vi "Intensity Graph Linecut (Horizontal).vi"(8 "error in (no error)":errorcluster, 9 "width (horizontal)":dbl, 11 "graph_utilities in":refnum<class "graph_utilities.lvclass">) -> (0 "error out":errorcluster, 3 "graph_utilities out":refnum<class "graph_utilities.lvclass">)   [LabVIEW 2016, in "graph_utilities.lvclass"]
uses:
  graph_utilities.lvclass
  <vilib>/Analysis/baseanly.llb/A x Vector.vi
  <vilib>/Analysis/NI_AALBase.lvlib
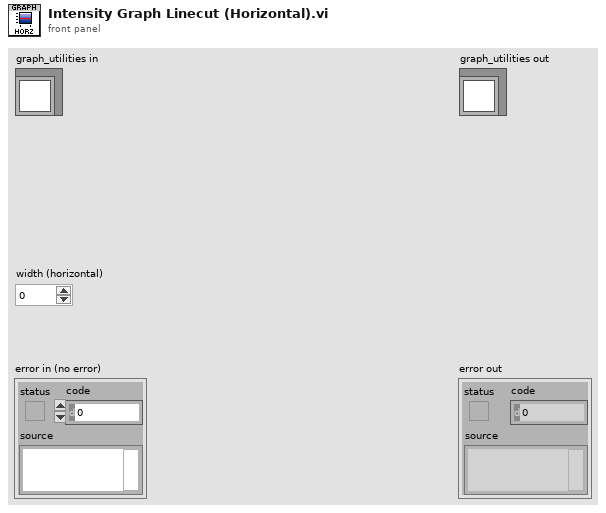
[diagram p1: front panel]
types:
  T1 = typedef "LVPointDoubleTypeDef.ctl" = cluster{"X":dbl, "Y":dbl}
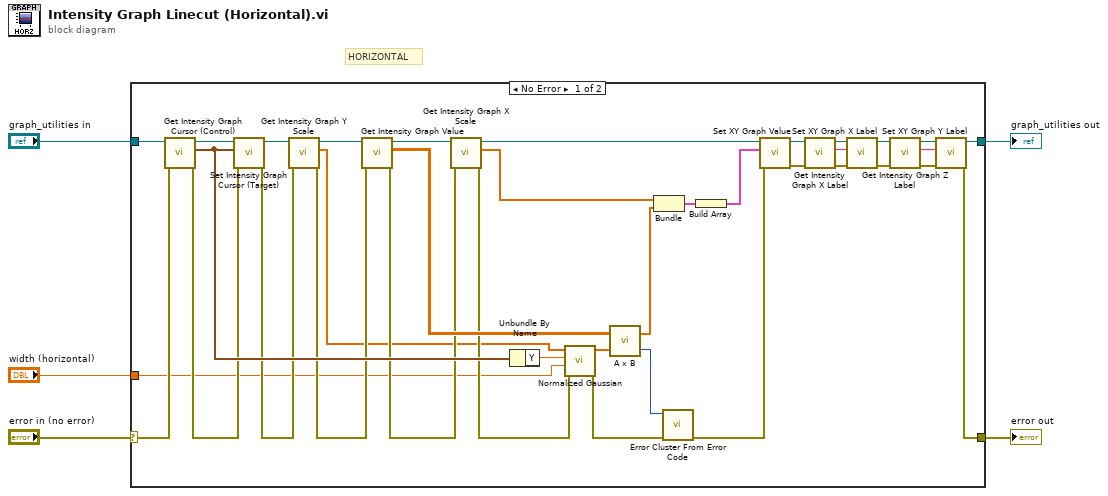
[diagram p0: block diagram]
diagram:
  # "HORIZONTAL"
  n1 = case shown="No Error" "error in (no error)" {
    selector: "error in (no error)" -> [w31 w44]
    tunnel: [w6 w44] -> w4
    tunnel: [w11 w43] -> w2
    tunnel: "graph_utilities in" -> [w33 w43]
    tunnel: "width (horizontal)" -> [w15 _]
    frame No Error {
      n2 = call "Get Intensity Graph Cursor (Control).vi"("error in (no error)"=w31, "graph_utilities in"=w33) -> ("error out"=w30:errorcluster, "Cursor.Cursor Position"=w35:T1, "graph_utilities out"=w34:refnum<class "graph_utilities.lvclass">)  [unwired: 7 in]
      n3 = call "Set Intensity Graph Cursor (Target).vi"("error in (no error)"=w30, "Cursor.Cursor Position"=w35, "graph_utilities in"=w34) -> ("error out"=w29:errorcluster, "graph_utilities out"=w32:refnum<class "graph_utilities.lvclass">)  [unwired: 7 in]
      n4 = call "Get Intensity Graph Y Scale.vi"("error in (no error)"=w29, "graph_utilities in"=w32) -> ("error out"=w28:errorcluster, "Y Scale"=w16:dbl[], "graph_utilities out"=w36:refnum<class "graph_utilities.lvclass">)  [unwired: 7 in]
      n5 = call "Get Intensity Graph Value.vi"("error in (no error)"=w28, "graph_utilities in"=w36) -> ("error out"=w27:errorcluster, "Value"=w38:dbl[][], "graph_utilities out"=w37:refnum<class "graph_utilities.lvclass">)  [unwired: 7 in]
      n6 = call "Get Intensity Graph X Scale.vi"("error in (no error)"=w27, "graph_utilities in"=w37) -> ("error out"=w26:errorcluster, "X Scale"=w39:dbl[], "graph_utilities out"=w17:refnum<class "graph_utilities.lvclass">)  [unwired: 7 in]
      n7 = Unbundle By Name(w35) -> ("Y"=w41:dbl)
      n8 = call "Normalized Gaussian.vi"("error in (no error)"=w26, "width (c)"=w15, "position (b)"=w41, "Scale"=w16) -> ("error out"=w25:errorcluster, "Normalized Gaussian"=w42:dbl[])  [unwired: 6 in]
      n9 = call-poly <vilib>:"A x B.vi"("Vector"=w42, "A"=w38) -> ("error"=w40:i32, "A x Vector"=w24:dbl[])
      n10 = Bundle("X Scale"=w39, "A x Vector"=w24) -> (w23:cluster{"X Scale":dbl[], "A x Vector":dbl[]})  [unwired: 1 in]
      n11 = call <vilib>:"Error Cluster From Error Code.vi"("error in (no error)"=w25, "error code (0)"=w40) -> ("error out"=w21:errorcluster)  [unwired: 7 in]
      n12 = Build Array(w23) -> (w22:cluster{"X Scale":dbl[], "A x Vector":dbl[]}[])
      n13 = call "Set XY Graph Value.vi"("error in (no error)"=w21, "Value"=w22, "graph_utilities in"=w17) -> ("error out"=w7:errorcluster, "graph_utilities out"=w14:refnum<class "graph_utilities.lvclass">)  [unwired: 7 in]
      n14 = call "Get Intensity Graph X Label.vi"("error in (no error)"=w7, "graph_utilities in"=w14) -> ("error out"=w20:errorcluster, "X Label"=w18:string, "graph_utilities out"=w19:refnum<class "graph_utilities.lvclass">)  [unwired: 7 in]
      n15 = call "Set XY Graph X Label.vi"("error in (no error)"=w20, "X Label"=w18, "graph_utilities in"=w19) -> ("error out"=w9:errorcluster, "graph_utilities out"=w10:refnum<class "graph_utilities.lvclass">)  [unwired: 7 in]
      n16 = call "Get Intensity Graph Z Label.vi"("error in (no error)"=w9, "graph_utilities in"=w10) -> ("error out"=w8:errorcluster, "Z Label"=w13:string, "graph_utilities out"=w12:refnum<class "graph_utilities.lvclass">)  [unwired: 7 in]
      n17 = call "Set XY Graph Y Label.vi"("error in (no error)"=w8, "Y Label"=w13, "graph_utilities in"=w12) -> ("error out"=w6:errorcluster, "graph_utilities out"=w11:refnum<class "graph_utilities.lvclass">)  [unwired: 7 in]
    }
    frame Error {
    }
  }
  "error out" <- w4
  "graph_utilities out" <- w2
